vi "Add Message.vi"(6 "ul_ByteCount":u32, 7 "ul_UdpHandle":u32, 8 "error in (no error)":errorcluster, 9 "index":i32, 10 "Message Block Array in":u32[](array[numeric]), 11 "Udp Block Message Map in":map{i32, T1}(c390)) -> (0 "error out":errorcluster, 2 "Message Block Array out":u32[](array[numeric]), 3 "Udp Block Message Map out":map{i32, T1}(c390))   [LabVIEW 2020, in "UdpBlockMessage.lvlib"]
uses:
  UdpBlockMessage.lvlib
  ubm_value_type.ctl
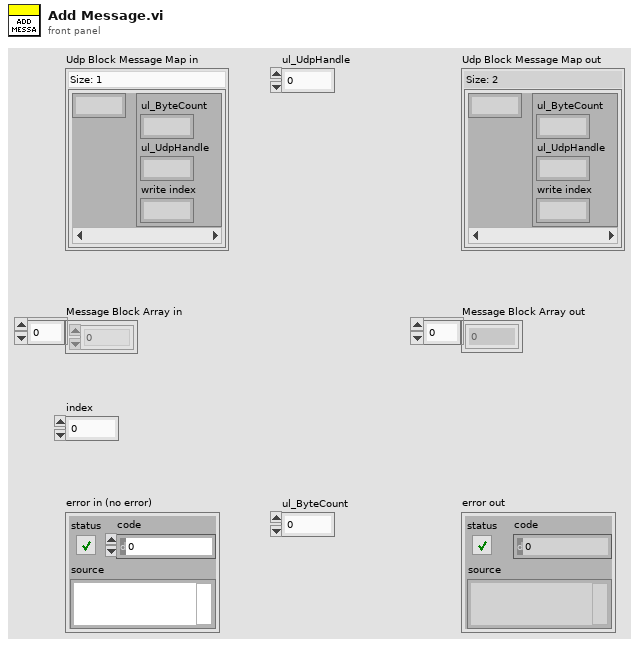
[diagram p1: front panel]
types:
  T1 = typedef "UdpBlockMessage.lvlib/ubm_value_type.ctl" = cluster{"ul_ByteCount":u32, "ul_UdpHandle":u32, "write index":u32}
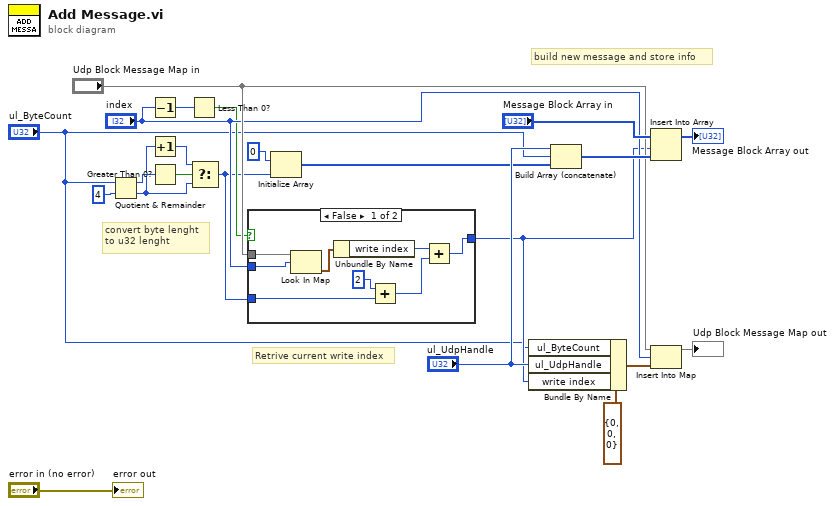
[diagram p0: block diagram]
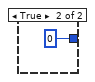
[diagram p2: hidden frame]
diagram:
  # "build new message and store info"
  # "Retrive current write index"
  # "convert byte lenght\nto u32 lenght"
  n1 = Quotient & Remainder(x="ul_ByteCount", y=u32 4) -> (x-y*floor(x/y)=w19:u32, floor(x/y)=w17:u32)
  n2 = Decrement(x="index") -> (x-1=w5:i32)
  n3 = Increment(x=w17) -> (x+1=w16:u32)
  n4 = Greater Than 0?(x=w19) -> (x > 0?=w18:bool)
  n5 = Less Than 0?(x=w5) -> (x < 0?=w4:bool)
  n6 = Select(t=w16, s=w18, f=w17) -> (s? t:f=w3:u32)
  n7 = case shown="False" w4 {
    tunnel: "Udp Block Message Map in" -> [w30 _]
    tunnel: "index" -> [w29 _]
    tunnel: w3 -> [w26 _]
    tunnel: [w23 u32 0 ("write index")] -> w2
    frame False {
      n8 = Look In Map(map=w30, key=w29) -> (value=w28:T1)  [unwired: 1 in, 1 out]
      n9 = Unbundle By Name(w28) -> ("write index"=w24:u32)
      n10 = Add(x=u32 2, y=w26) -> (x+y=w27:u32)
      n11 = Add(x=w24, y=w27) -> (x+y=w23:u32)
    }
    frame True {
    }
  }
  n12 = Initialize Array(u32 0 ("y"), w3) -> (w13:u32[])
  n13 = Bundle By Name(cluster=T1 {"ul_ByteCount"=0, "ul_UdpHandle"=0, "write index"=0} ("value"), "ul_ByteCount"="ul_ByteCount", "ul_UdpHandle"="ul_UdpHandle", "write index"=w2) -> (w21:T1)
  n14 = Build Array (concatenate)("ul_UdpHandle", "ul_ByteCount", w13) -> (w11:u32[])
  n15 = Insert Into Array(array="Message Block Array in", index=w2, new element=w11) -> (→"Message Block Array out":u32[])
  n16 = Insert Into Map(map in="Udp Block Message Map in", key="index", value=w21) -> (map out=→"Udp Block Message Map out":map{i32, T1})  [unwired: 2 out]
  "error out" <- "error in (no error)"
